vi "Packager Output Files Path.vi"(0 "Project Path":path) -> (4 "Package Path":path, 6 "Build Outputs Path":path)   [LabVIEW 2021, in "Path Functions.lvlib"]
uses:
  Path Functions.lvlib
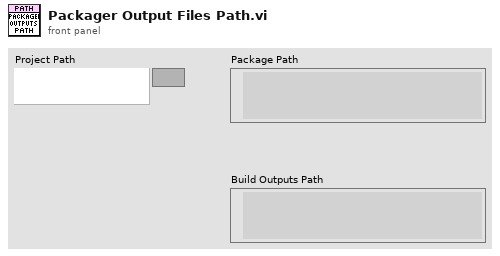
[diagram p1: front panel]
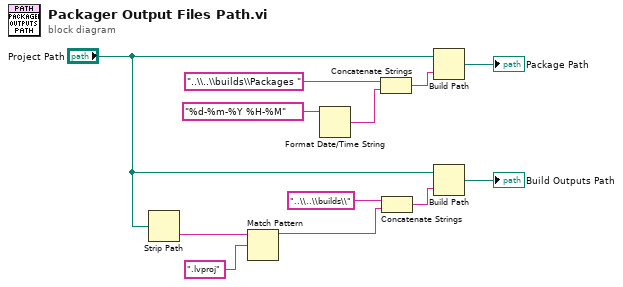
[diagram p0: block diagram]
diagram:
  n1 = Strip Path(path="Project Path") -> (name=w10:string)  [unwired: 1 out]
  n2 = Match Pattern(string=w10, regular expression=".lvproj") -> (before substring=w9:string)  [unwired: 1 in, 3 out]
  n3 = Format Date/Time String(time format string (%c)="%d-%m-%Y %H-%M") -> (date/time string=w8:string)  [unwired: 2 in]
  n4 = Concatenate Strings("..\\..\\builds\\Packages ", w8) -> (w4:string)
  n5 = Concatenate Strings("..\\..\\builds\\", w9) -> (w5:string)
  n6 = Build Path(base path="Project Path", name or relative path=w4) -> (appended path=→"Package Path":path)
  n7 = Build Path(base path="Project Path", name or relative path=w5) -> (appended path=→"Build Outputs Path":path)
